vi "Write TCP Configs.vi"(8 "error in (no error)":errorcluster, 10 "Item Ref in":T1 format="%.0x", 11 "Refnum in":T2) -> (0 "error out":errorcluster, 2 "Item Ref out":T1 format="%.0x", 3 "Refnum out":T2)   [LabVIEW 2020, in "Modbus Master System Explorer.lvlib"]
uses:
  Modbus Master System Explorer.lvlib
  <vilib>/Utility/config.llb/Config Data RefNum.ctl
  <vilib>/NI VeriStand/Custom Device API/Custom Device Item Ref.ctl
  <vilib>/Utility/config.llb/Write Key (String).vi
  <vilib>/Utility/config.llb/Write Key (U32).vi
  <vilib>/Utility/config.llb/NI_LVConfig.lvlib
  <vilib>/NI VeriStand/Custom Device API/Custom Device API.lvlib
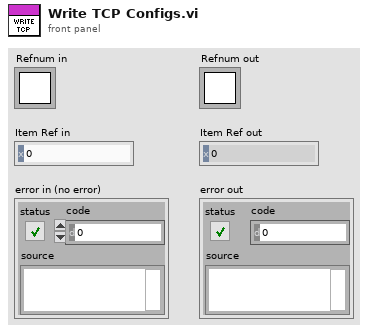
[diagram p1: front panel]
types:
  T1 = typedef "Custom Device API.lvlib/Custom Device Item Ref.ctl" = u64
  T2 = typedef "NI_LVConfig.lvlib/Config Data RefNum.ctl" = refnum<k1>
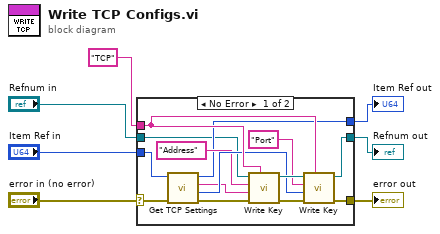
[diagram p0: block diagram]
diagram:
  n1 = case shown="No Error" "error in (no error)" {
    selector: "error in (no error)" -> [w9 w23]
    tunnel: [w21 w23] -> w7
    tunnel: [w20 w24] -> w6
    tunnel: "TCP" ("section") -> [w18 _]
    tunnel: [w11 w22] -> w4
    tunnel: "Refnum in" -> [w10 w24]
    tunnel: "Item Ref in" -> [w8 w22]
    frame No Error {
      n2 = call "Get TCP Settings.vi"("error in (no error)"=w9, "Item Ref in"=w8) -> ("error out"=w17:errorcluster, "Port"=w15:u16, "Address"=w13:string, "Item Ref out"=w11:T1)  [unwired: 5 in, 1 out]
      n3 = call-poly <vilib>:"Write Key.vi"("section"=w18, "error in (no error)"=w17, "value"=w13, "key"="Address", "refnum"=w10) -> ("error out"=w16:errorcluster, "refnum out"=w19:T2)  [unwired: 4 in, 1 out]
      n4 = call-poly <vilib>:"Write Key.vi"("section"=w18, "error in (no error)"=w16, "value"=w15, "key"="Port", "refnum"=w19) -> ("error out"=w21:errorcluster, "refnum out"=w20:T2)  [unwired: 4 in, 1 out]
    }
    frame Error {
    }
  }
  "error out" <- w7
  "Refnum out" <- w6
  "Item Ref out" <- w4
